vi "Export2SheetString.vi"(6 "波形数组":cluster{dbl[], dbl[]}[](array[cluster]), 9 "信号名数组":string[](array[string]), 10 "进度数值":refnum<vi>, 11 "Slide输入":refnum<vi>) -> (3 "SheetSpread":string[][](array[string]))   [LabVIEW 2015]
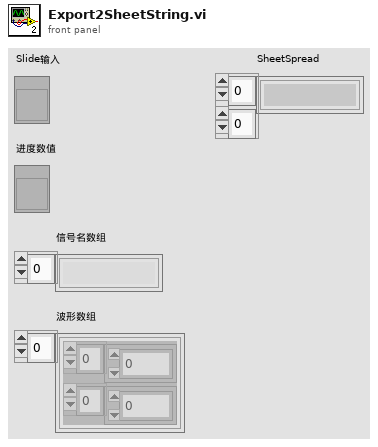
[diagram p1: front panel]
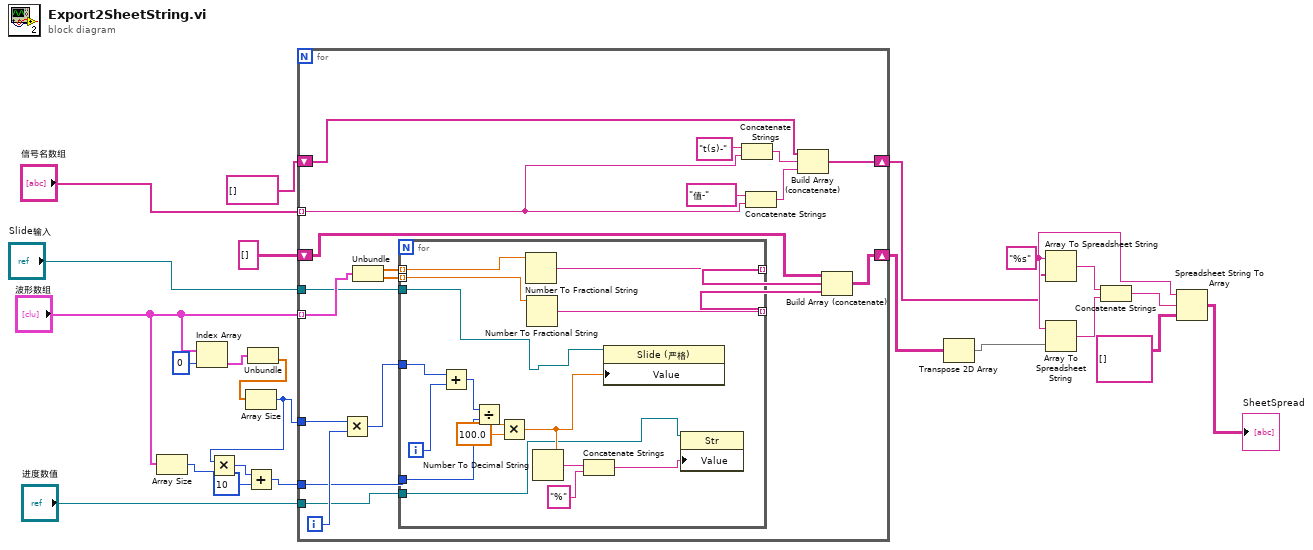
[diagram p0: block diagram]
diagram:
  w20 = "%s" ("格式字符串")
  n1 = Array Size(array="波形数组") -> (size(s)=w9:i32)
  n2 = Index Array(array="波形数组", index=0 ("索引")) -> (element=w7:cluster{dbl[], dbl[]})
  n3 = Unbundle(w7) -> (w8:dbl[])  [unwired: 1 out]
  n4 = Array Size(array=w8) -> (size(s)=w10:i32)
  n5 = Multiply(x=w10, y=w9) -> (x*y=w11:i32)
  n6 = Add(x=w11, y=10) -> (x+y=w12:i32)
  n7 = for {
    tunnel: "波形数组" -> [w39] mode=indexing
    shift-right: [w38] -> w3
    shift-left: string[][] [] -> [w37]
    tunnel: "信号名数组" -> [w33] mode=indexing
    shift-right: [w31] -> w14
    shift-left: string[] [] -> [w30]
    tunnel: w10 -> [w28]
    tunnel: w12 -> [w26]
    tunnel: "Slide输入" -> [w25]
    tunnel: "进度数值" -> [w24]
    i -> [w29]
    n8 = Multiply(x=w28, y=w29) -> (x*y=w27:i32)
    n9 = Unbundle(w39) -> (w43:dbl[], w42:dbl[])
    n10 = for {
      tunnel: w43 -> [w59] mode=indexing
      tunnel: w42 -> [w57] mode=indexing
      tunnel: [w58] -> w41 mode=indexing
      tunnel: [w56] -> w40 mode=indexing
      tunnel: w27 -> [w55]
      tunnel: w26 -> [w52]
      tunnel: w25 -> [w45]
      tunnel: w24 -> [w44]
      i -> [w54]
      n11 = Add(x=w55, y=w54) -> (x+y=w53:i32)
      n12 = Divide(x=w53, y=w52) -> (x/y=w51:dbl)
      n13 = Multiply(x=w51, y=100.0) -> (x*y=w46:dbl)
      n14 = Number To Fractional String(number=w59) -> (F-format string=w58:string)  [unwired: 3 in]
      n15 = Number To Fractional String(number=w57) -> (F-format string=w56:string)  [unwired: 3 in]
      n16 = Number To Decimal String(number=w46) -> (decimal integer string=w49:string)  [unwired: 1 in]
      n17 = Concatenate Strings(w49, "%" ("字符串")) -> (w47:string)
      n18 = property class="Slide (严格)"(reference=w45, "Value"=w46) -> ()  [unwired: 1 in, 2 out]
      n19 = property class="Str"(reference=w44, "Value"=w47) -> ()  [unwired: 1 in, 2 out]
    }
    n20 = Concatenate Strings("t(s)-" ("字符串"), w33) -> (w36:string)
    n21 = Concatenate Strings("值-" ("字符串"), w33) -> (w32:string)
    n22 = Build Array (concatenate)(w30, w36, w32) -> (w31:string[])
    n23 = Build Array (concatenate)(w37, w41, w40) -> (w38:string[][])
  }
  n24 = Transpose 2D Array(2D array=w3) -> (transposed array=w15:string[][])
  n25 = Array To Spreadsheet String(array=w14, 3:w20) -> (spreadsheet string=w16:string)  [unwired: 1 in]
  n26 = Array To Spreadsheet String(array=w15, 3:w20) -> (spreadsheet string=w17:string)  [unwired: 1 in]
  n27 = Concatenate Strings(w16, w17) -> (w18:string)
  n28 = Spreadsheet String To Array(format string=w20, spreadsheet string=w18, array type (2D Dbl)=string[][] []) -> (array=→"SheetSpread":string[][])  [unwired: 1 in]
